vi "setUp.vi"(8 "error in (no error)":errorcluster, 11 "VI in":refnum<vi>) -> (0 "error out":errorcluster, 3 "fpMgr out":refnum<class "VIProviderShellHelper.lvclass">)   [LabVIEW 2019, in "LabVIEW-ProviderShell.lvlib" / "VIProviderShellHelper.lvclass"]
uses:
  VIProviderShellHelper.lvclass
  Support/def-ConnectorInfo.ctl
  VIProviderShellHelper.lvclass/VIProviderShellHelper.ctl
  fd6465c0-90c1-4b18-8ed0-c20eb5624f43.vi
  e0c14180-a7ac-40a3-8398-1e950974c387.vi
  LabVIEW-ProviderShell.lvlib
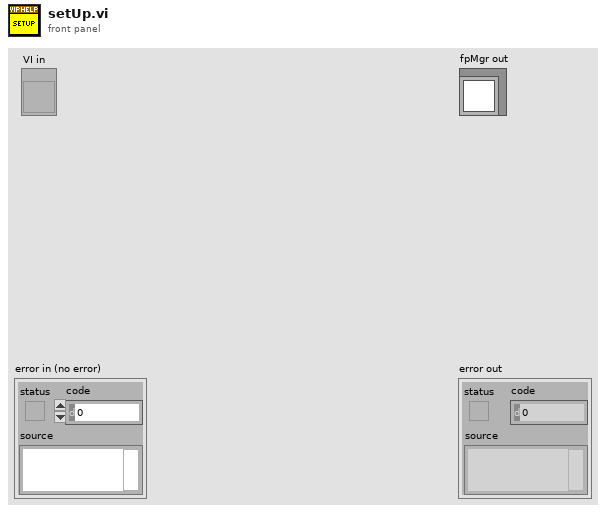
[diagram p1: front panel]
types:
  T1 = typedef "LabVIEW-ProviderShell.lvlib/VIProviderShellHelper.lvclass/def-ConnectorInfo.ctl" = cluster{"Value":variant, "Label.Text":string, "error":errorcluster, "DatatypeDescription":string, "Indicator":bool}
  T2 = typedef "Type Descriptor__ogtk.ctl" = i16[]
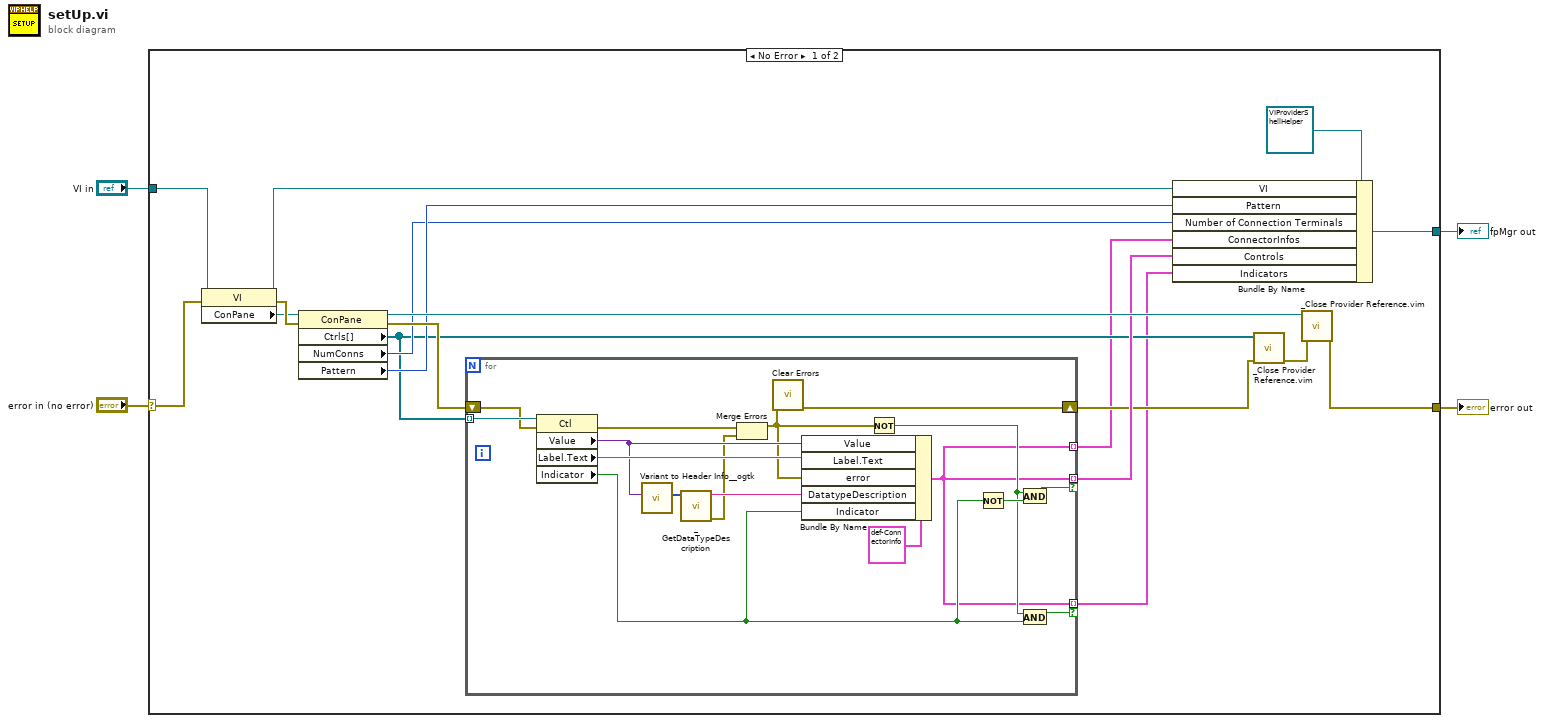
[diagram p0: block diagram]
diagram:
  n1 = case shown="No Error" "error in (no error)" {
    selector: "error in (no error)" -> [w19 w40]
    tunnel: [w21 w40] -> w3
    tunnel: "VI in" -> [w16 _]
    tunnel: [w10 _] -> w1
    frame No Error {
      n2 = property on="Property Node" class="VI"(reference=w16, error in=w19) -> (reference out=w14:refnum<vi>, error out=w18:errorcluster, "ConPane"=w17:refnum<vi>)
      n3 = property on="Property Node" class="ConPane"(reference=w17, error in=w18) -> (reference out=w22:refnum<vi>, error out=w20:errorcluster, "Ctrls[]"=w9:refnum<vi>[], "NumConns"=w11:u32, "Pattern"=w12:u32)
      n4 = for {
        tunnel: w9 -> [w39] mode=indexing
        shift-right: [w37] -> w7
        shift-left: w20 -> [w38]
        tunnel: [w25] -> w13 mode=indexing if=w28
        tunnel: [w25] -> w6 mode=indexing if=w29
        tunnel: [w25] -> w5 mode=indexing
        n5 = property class="Ctl"(reference=w39, error in=w38) -> (error out=w34:errorcluster, "Value"=w33:variant, "Label.Text"=w35:string, "Indicator"=w31:bool)  [unwired: 1 out]
        n6 = call <userlib>:"Variant to Header Info__ogtk.vi"("Variant"=w33) -> ("Type Descriptor"=w24:T2)  [unwired: 3 in, 2 out]
        n7 = call "_GetDataTypeDescription.vi"("Type Descriptor"=w24) -> ("error out"=w23:errorcluster, "String"=w32:string)  [unwired: 9 in]
        n8 = Merge Errors(w34, w23) -> (w27:errorcluster)
        n9 = call <vilib>:"Clear Errors.vi"("error in (no error)"=w27) -> ("error out"=w37:errorcluster)  [unwired: 5 in, 1 out]
        n10 = Bundle By Name(cluster=T1 {"Value"=variant, "Label.Text"="", "error"={"status"=FALSE, "code"=0, "source"=""}, "DatatypeDescription"="", "Indicator"=FALSE} ("Cluster"), "Value"=w33, "Label.Text"=w35, "error"=w27, "DatatypeDescription"=w32, "Indicator"=w31) -> (w25:T1)
        n11 = Not(x=w27) -> (.not. x?=w26:bool)
        n12 = Not(x=w31) -> (.not. x?=w30:bool)
        n13 = And(x=w26, y=w30) -> (x .and. y?=w28:bool)
        n14 = And(x=w26, y=w31) -> (x .and. y?=w29:bool)
      }
      n15 = Bundle By Name(cluster=refnum<class "VIProviderShellHelper.lvclass"> refnum ("LabVIEW-ProviderShell.lvlib:fpMgr.lvclass"), "VI"=w14, "Pattern"=w12, "Number of Connection Terminals"=w11, "ConnectorInfos"=w5, "Controls"=w13, "Indicators"=w6) -> (w10:refnum<class "VIProviderShellHelper.lvclass">)
      n16 = call "_Close Provider Reference.vim"("error in (no error)"=w7, "LVClassLibrary in"=w9) -> ("error out"=w8:errorcluster)  [unwired: 9 in]
      n17 = call "_Close Provider Reference.vim"("error in (no error)"=w8, "LVClassLibrary in"=w22) -> ("error out"=w21:errorcluster)  [unwired: 9 in]
    }
    frame Error {
    }
  }
  "error out" <- w3
  "fpMgr out" <- w1
